vi "Is Full Errors.vi"(8 "error in (no error)":errorcluster, 11 "Session in":refnum<class "Session.lvclass">) -> (0 "error out":errorcluster, 2 "Full Errors":bool, 3 "Session out":refnum<class "Session.lvclass">)   [LabVIEW 2020, in "CTI.lvlib" / "Session.lvclass"]
uses:
  Session.lvclass
  Session.lvclass/Session.ctl
  Error Reporting.ctl
  CTI.lvlib
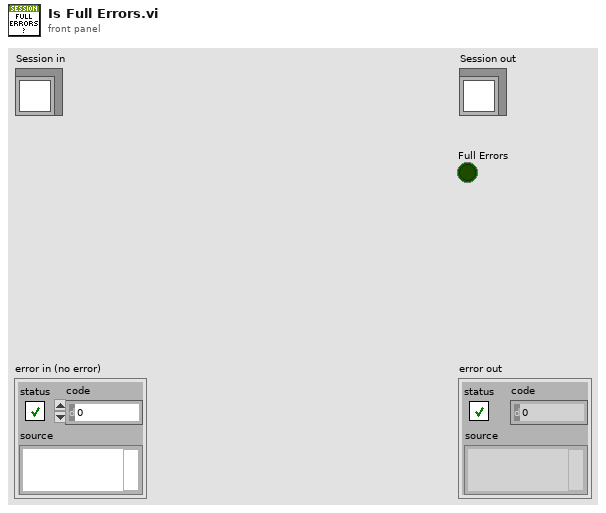
[diagram p1: front panel]
types:
  T1 = typedef "CTI.lvlib/Error Reporting.ctl" = enum16{"Minimal", "Moderate", "Full"}
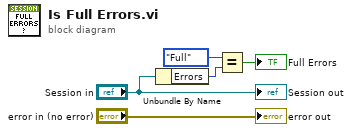
[diagram p0: block diagram]
diagram:
  n1 = Unbundle By Name("Session in") -> ("Errors"=w3:T1)
  n2 = Equal?(x=Error_Reporting."Full", y=w3) -> (x = y?=→"Full Errors":bool)
  "error out" <- "error in (no error)"
  "Session out" <- "Session in"
